vi "Run.vi"(8 "error in (no error)":errorcluster, 11 "RoomAlert in":refnum<class "RoomAlert.lvclass">) -> (0 "error out":errorcluster, 1 "DataValid":bool, 2 "clSensorData":T1, 3 "RoomAlert out":refnum<class "RoomAlert.lvclass">)   [LabVIEW 2018, in "SensorPlugins.lvlib" / "RoomAlert.lvclass"]
doc: "Retrieves measurements from the RoomAlert instrument."
uses:
  RoomAlert.lvclass
  SensorShared/clSensorData.ctl
  SensorShared/SensorVisulization.ctl
  <vilib>/Utility/error.llb/Error Cluster From Error Code.vi
  <vilib>/ErrorRing/Error Ring.xnode
  SensorShared/SensorShared.lvlib
panel:
  out "Execution Time (ms)":u32
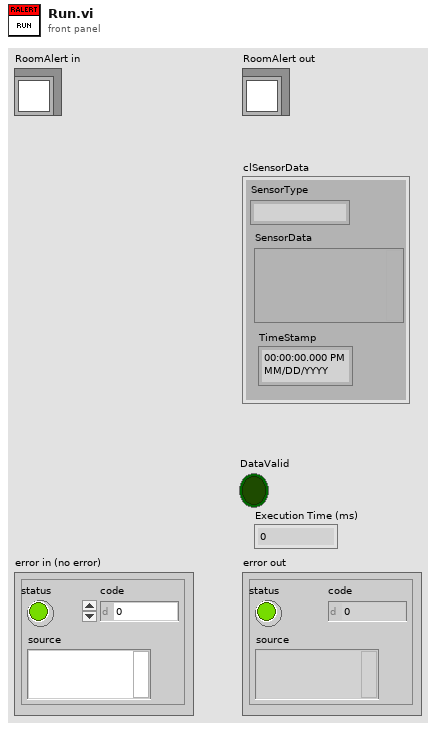
[diagram p1: front panel]
types:
  T1 = typedef "SensorShared.lvlib/clSensorData.ctl" = cluster{"SensorType":string, "SensorData":variant, "TimeStamp":timestamp}
  T2 = typedef "SensorShared.lvlib/SensorVisulization.ctl" = cluster{"Array of Waveforms":waveform(dbl)[], "Array of Strings ":string[], "LightTower":cluster{"Red":bool, "Amber":bool, "Green":bool, "Audio":bool}}
  T3 = typedef "SensorPlugins.lvlib/RoomAlert.lvclass/RoomAlertControls.ctl" = cluster{"Connected?":bool, "IP Address of SNMP Device":string, "Port (161)":u16, "Community Name":string, "Measurements To Read Array":u16[], "Update LightTower?":bool, "LightTower":cluster{"Red":bool, "Amber":bool, "Green":bool, "Audio":bool}, "RoomAlert Model ID":string, "Sensor OID Numbers":string[][], "Sensor Light Tower OID Numbers":string[][]}[]
  T4 = typedef "SensorPlugins.lvlib/RoomAlert.lvclass/CommunicationControls.ctl" = refnum<k16>[]
  T5 = typedef "SensorPlugins.lvlib/RoomAlert.lvclass/MeasurementControls.ctl" = cluster{"Measurement RefreshTime (ms)":u32, "Measurement Name":string, "Timeout(ms)":i32, "Amber Warning Light Configuration":cluster{"Warning Temperture (Degrees C)":dbl, "Temperature Delta (Degrees C/Minute)":dbl, "Time Window (Minutes)":dbl}}
  T6 = cluster{"Warning Temperture (Degrees C)":dbl, "Temperature Delta (Degrees C/Minute)":dbl, "Time Window (Minutes)":dbl}
  T7 = cluster{"[0]":bool, "[1]":bool, "[2]":bool, "[3]":bool}
  T8 = cluster{"Connected?":bool, "IP Address of SNMP Device":string, "Port (161)":u16, "Community Name":string, "Measurements To Read Array":u16[], "Update LightTower?":bool, "LightTower":cluster{"Red":bool, "Amber":bool, "Green":bool, "Audio":bool}, "RoomAlert Model ID":string, "Sensor OID Numbers":string[][], "Sensor Light Tower OID Numbers":string[][]}
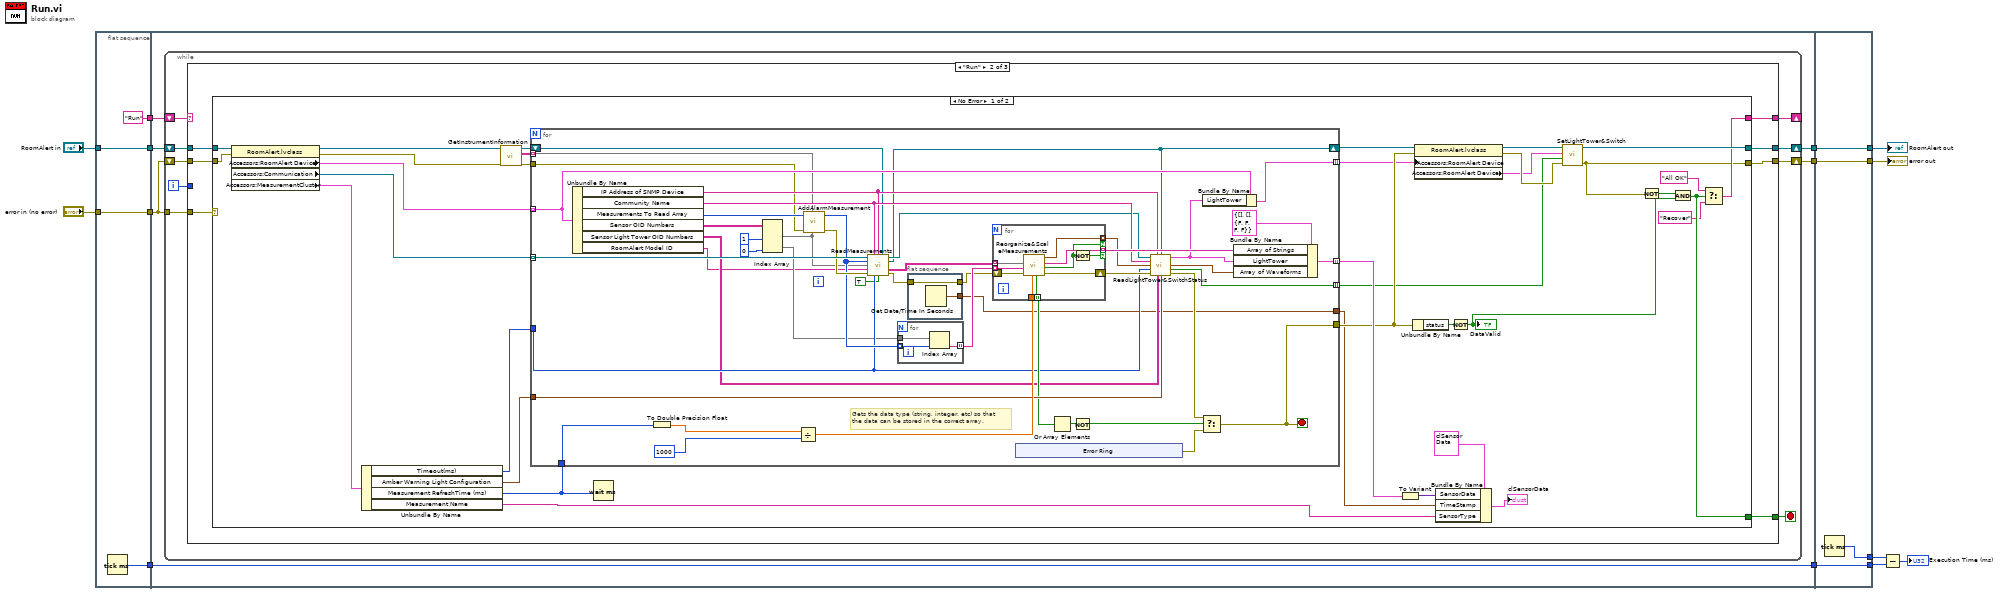
[diagram p0: block diagram]
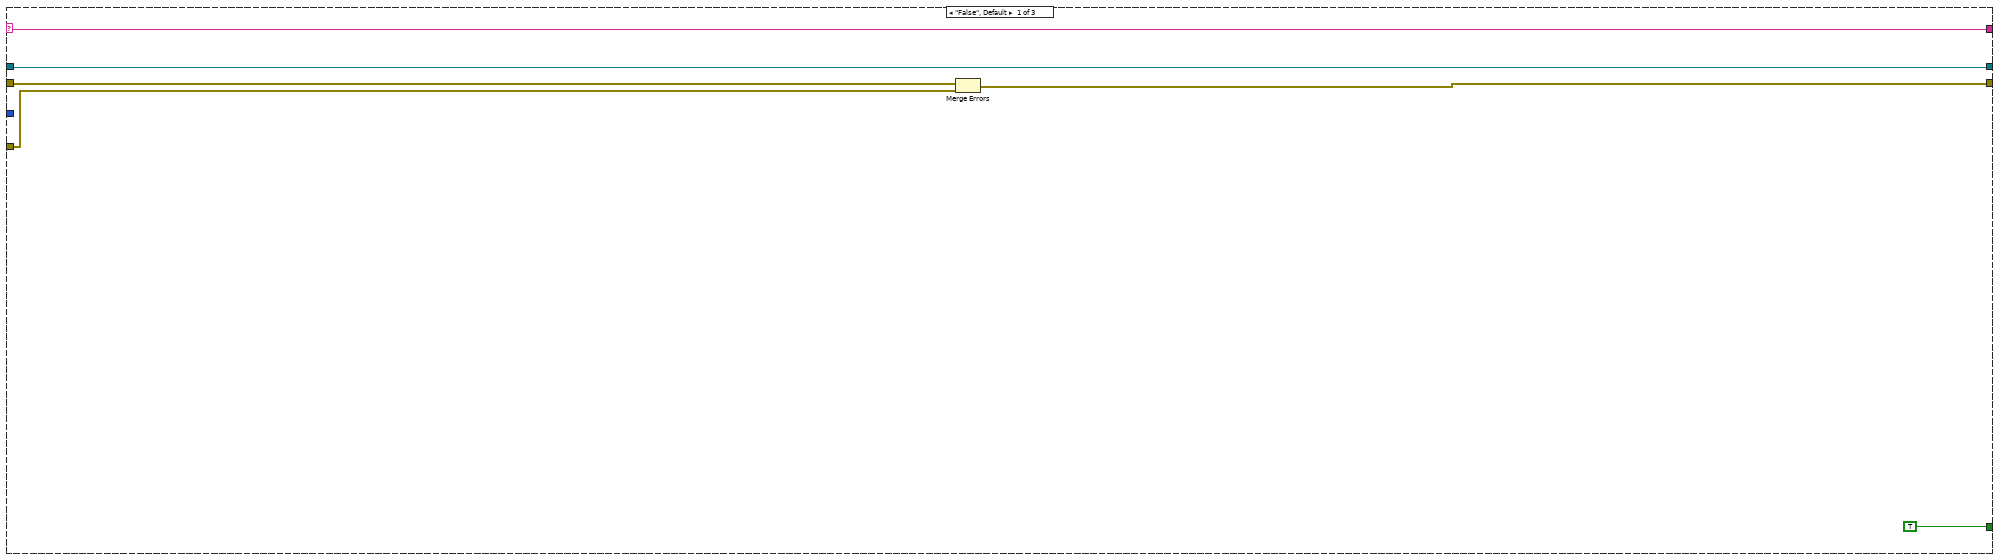
[diagram p2: hidden frame]
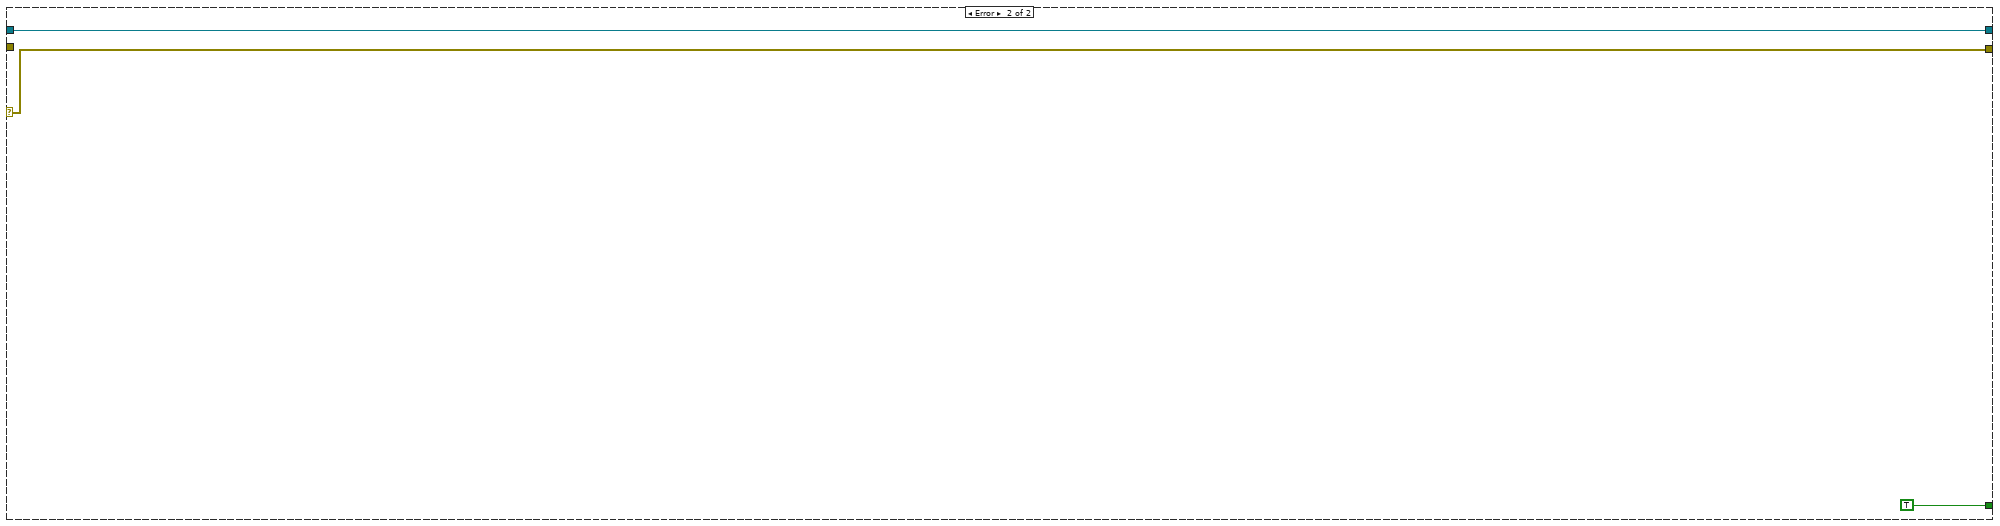
[diagram p3: hidden frame]
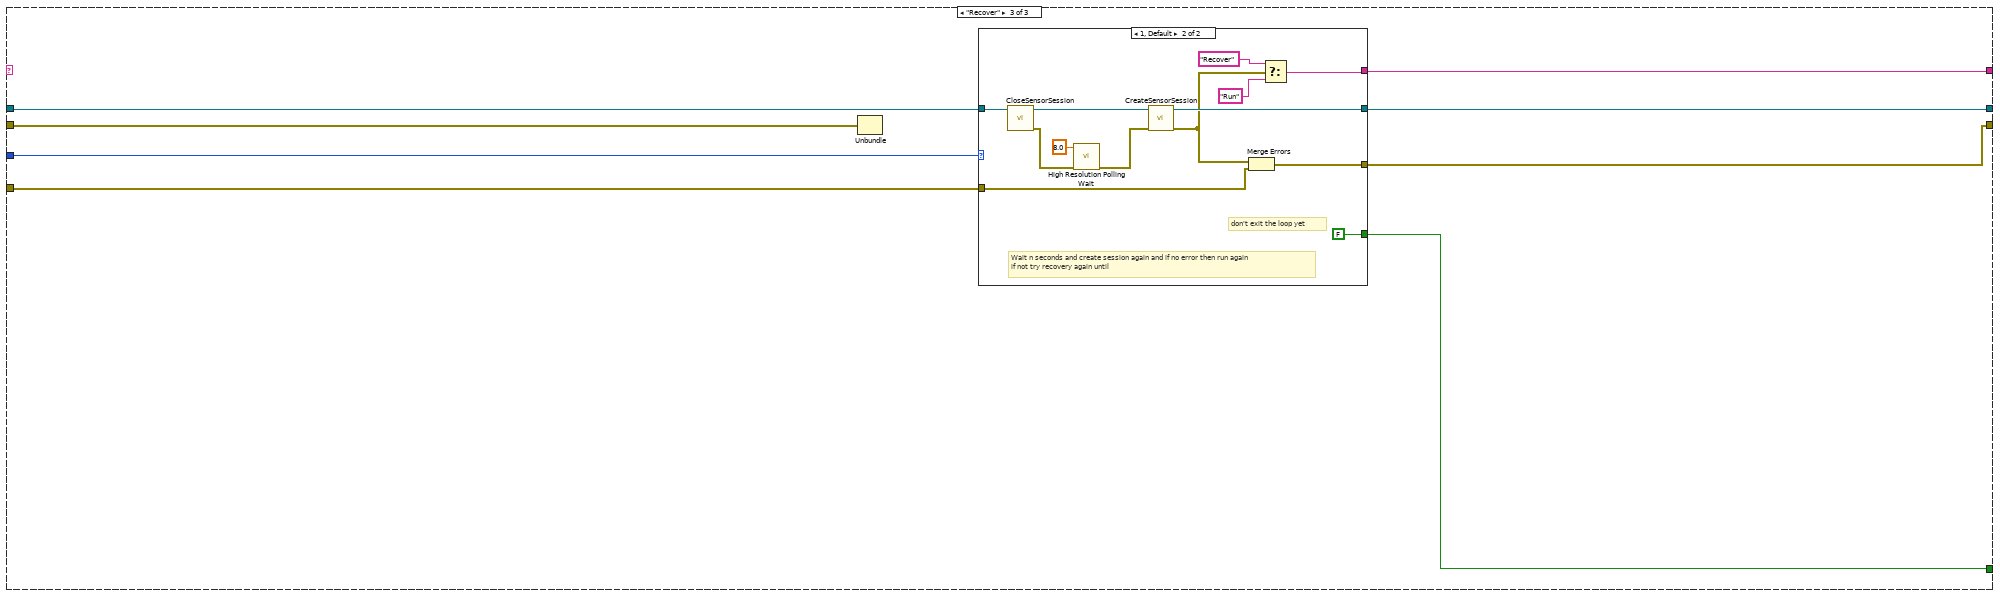
[diagram p4: hidden frame]
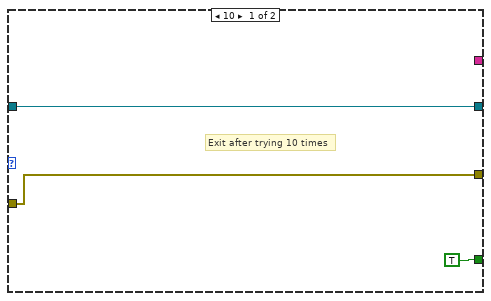
[diagram p5: hidden frame]
diagram:
  n1 = flat-sequence {
    tunnel: "RoomAlert in" -> [w17]
    tunnel: "error in (no error)" -> [w18]
    tunnel: [w18] -> w14
    tunnel: [w17] -> w13
    tunnel: [w16] -> w12
    tunnel: ["Run" ("Measurement Name")] -> w1
    tunnel: w14 -> [w19]
    tunnel: w13 -> [w24]
    tunnel: [w23] -> w9
    tunnel: [w22] -> w10
    tunnel: w12 -> [w21]
    tunnel: [w21] -> w11
    tunnel: w1 -> [w20]
    tunnel: [w177] -> w5
    tunnel: [w178] -> w6
    tunnel: w11 -> [w175]
    tunnel: w10 -> [w177]
    tunnel: w9 -> [w178]
    tunnel: [w176] -> w3
    tunnel: [w175] -> w2
    frame #0 {
      n2 = Tick Count (ms)() -> (millisecond timer value=w16:u32)
    }
    frame #1 {
      n3 = while {
        shift-right: [w30] -> w22
        shift-left: w19 -> [w33]
        shift-right: [w31] -> w23
        shift-left: w24 -> [w32]
        shift-right: [w28] -> _
        shift-left: w20 -> [w29]
        tunnel: w19 -> [w26]
        i -> [w25]
        stop <- w27 stop-if-true
        n4 = case shown="\"Run\"" w29 {
          selector: w29 -> [w39 _ _]
          tunnel: w33 -> [w37 w40 w151]
          tunnel: w32 -> [w38 w46 w158]
          tunnel: [w38 w45 w157] -> w31
          tunnel: [w36 w44 w153] -> w30
          tunnel: [w39 w43 w156] -> w28
          tunnel: [TRUE w42 w154] -> w27
          tunnel: w26 -> [w35 w41 w152]
          tunnel: w25 -> [_ _ w155]
          frame "False", Default {
            n5 = Merge Errors(w37, w35) -> (w36:errorcluster)
          }
          frame "Run" {
            n6 = case shown="No Error" w41 {
              selector: w41 -> [_ w150]
              tunnel: w46 -> [w81 w149]
              tunnel: [w52 w150] -> w44
              tunnel: [w69 w149] -> w45
              tunnel: [w55 _] -> w43
              tunnel: [w54 TRUE] -> w42
              tunnel: w40 -> [w53 _]
              frame No Error {
                n7 = property class="RoomAlert.lvclass"(reference=w81, error in=w53) -> (reference out=w65:refnum<class "RoomAlert.lvclass">, error out=w63:errorcluster, "Accessors:RoomAlert Device"=w57:T3, "Accessors:Communication "=w75:T4, "Accessors:MeasurementCluster"=w74:T5)
                n8 = Unbundle By Name(w74) -> ("Timeout(ms)"=w59:i32, "Amber Warning Light Configuration"=w58:T6, "Measurement RefreshTime (ms)"=w60:u32, "Measurement Name"=w48:string)
                n9 = call "GetInstrumentInformation.vi"("error in (no error)"=w63, "RoomAlert in"=w65) -> ("error out"=w62:errorcluster, "Model IDs"=w61:string[][][], "RoomAlert out"=w64:refnum<class "RoomAlert.lvclass">)  [unwired: 7 in]
                n10 = for {
                  tunnel: w57 -> [w101] mode=indexing
                  tunnel: [w111] -> w72
                  tunnel: [w127] -> w77 mode=indexing
                  tunnel: w75 -> [w126] mode=indexing
                  tunnel: w58 -> [w116]
                  tunnel: [w109] -> w68 mode=indexing
                  shift-right: [w85] -> w73
                  shift-left: w64 -> [w86]
                  tunnel: [w103] -> w66 mode=indexing
                  tunnel: w62 -> [w95]
                  tunnel: w61 -> [w98] mode=indexing
                  tunnel: w59 -> [w97]
                  tunnel: w60 -> [w96]
                  tunnel: [w82] -> w47
                  stop <- w111 stop-if-true
                  # "Gets the data type (string, integer, etc) so that\nthe data can be stored in the correct array."
                  n11 = Unbundle By Name(w101) -> ("IP Address of SNMP Device"=w118:string, "Community Name"=w119:string, "Measurements To Read Array"=w102:u16[], "Sensor OID Numbers"=w94:string[][], "Sensor Light Tower OID Numbers"=w89:string[][], "RoomAlert Model ID"=w87:string)
                  n12 = To Double Precision Float(number=w96) -> (double precision float=w124:dbl)
                  n13 = Index Array(array=w94, index (col) #1=1 ("disabled index (col)"), index (col) #2=0 ("index (col)")) -> (element #1=w92:string[], element #2=w90:string[])  [unwired: 2 in]
                  n14 = Divide(x=w124, y=u32 1000) -> (x/y=w122:dbl)
                  n15 = call "AddAlarmMeasurement.vi"("OID Numbers"=w92, "Model Information"=w98, "Error In"=w95, "Measurements To Read Array In"=w102) -> ("Error Out"=w100:errorcluster, "Measurements To Read Array Out"=w99:u16[])  [unwired: 6 in]
                  n16 = call "ReadMeasurements.vi"("UDP Network Connection in"=w126, "Community Name"=w119, "IP Address of SNMP Device"=w118, "RoomAlert in"=w86, "Measurements To Read Array"=w99, "OID Numbers"=w92, "Instrument Model ID"=w87, "error in (no error)"=w100, "Timeout(ms)"=w97, "Filter OID Numbers? (T)"=TRUE) -> ("UDP Network Connection out"=w106:refnum<k16>, "RoomAlert Out"=w85:refnum<class "RoomAlert.lvclass">, "SNMPDataAsStrings"=w117:string[][], "error out"=w84:errorcluster)  [unwired: 2 in]
                  n17 = for {
                    tunnel: w99 -> [w136] mode=indexing
                    tunnel: w90 -> [w137]
                    tunnel: [w135] -> w120 mode=indexing
                    n18 = Index Array(array=w137, index=w136) -> (element=w135:string)
                  }
                  n19 = flat-sequence {
                    tunnel: w84 -> [w129]
                    tunnel: [w129] -> w83
                    tunnel: [w128] -> w82
                    frame #0 {
                      n20 = Get Date/Time In Seconds() -> (seconds since 1Jan1904=w128:timestamp)
                    }
                  }
                  n21 = for {
                    tunnel: w117 -> [w138] mode=indexing
                    shift-right: [w146] -> w108
                    shift-left: w83 -> [w147]
                    tunnel: [w145] -> w105 mode=indexing if=w142
                    tunnel: w122 -> [w141]
                    tunnel: [w144] -> w123 mode=indexing if=w143
                    tunnel: w120 -> [w139] mode=indexing
                    tunnel: [w140] -> w115 mode=indexing
                    n22 = call "Reorganize&ScaleMeasurements.vi"("Meas Aperature"=w141, "Error In"=w147, "MeasurementType"=w139, "SNMPDataAsStrings"=w138) -> ("Error Out"=w146:errorcluster, "Numerical Information"=w142:bool, "String Data"=w144:string, "output waveform"=w145:waveform(dbl), "Alarmed"=w140:bool)  [unwired: 3 in]
                    n23 = Not(x=w142) -> (.not. x?=w143:bool)
                  }
                  n24 = xnode "Error Ring"() -> ("error out"=w114:errorcluster)
                  n25 = Or Array Elements(Boolean array=w115) -> (logical OR=w113:bool)
                  n26 = Not(x=w113) -> (.not. x?=w112:bool)
                  n27 = call "ReadLightTower&SwitchStatus.vi"("UDP Network Connection in"=w106, "IP Address of SNMP Device"=w118, "RoomAlert in"=w85, "Community Name"=w119, "Array In"=w105, "Timeout(ms)"=w97, "error in (no error)"=w108, "LightTower OID"=w89, "Amber Warning Light Limits"=w116) -> ("Light Tower"=w110:T7, "Array Out"=w104:waveform(dbl)[], "Yellow Limit Exceeded?"=w103:bool, "error out"=w107:errorcluster)  [unwired: 3 in]
                  n28 = Select(t=w107, s=w112, f=w114) -> (s? t:f=w111:errorcluster)
                  n29 = Bundle By Name(cluster=w101, "LightTower"=w110) -> (w109:T8)
                  n30 = Bundle By Name(cluster=T2 {"Array of Waveforms"=[], "Array of Strings "=[], "LightTower"={"Red"=FALSE, "Amber"=FALSE, "Green"=FALSE, "Audio"=FALSE}} ("SiemensDEMMeasurements 2"), "Array of Strings"=w123, "LightTower"=w110, "Array of Waveforms"=w104) -> (w127:T2)
                }
                n31 = Wait (ms)(milliseconds to wait=w60) -> ()  [unwired: 1 out]
                n32 = To Variant(anything=w77) -> (Variant=w79:variant)
                n33 = Unbundle By Name(w72) -> ("status"=w78:bool)
                n34 = property class="RoomAlert.lvclass"(reference=w73, error in=w72, "Accessors:RoomAlert Device"=w68) -> (reference out=w70:refnum<class "RoomAlert.lvclass">, error out=w71:errorcluster, "Accessors:RoomAlert Device"=w67:T3)
                n35 = Bundle By Name(cluster=T1 {"SensorType"="", "SensorData"=variant, "TimeStamp"=timestamp(0 s since 1904-01-01)} ("clSensorData"), "SensorData"=w79, "TimeStamp"=w47, "SensorType"=w48) -> (→"clSensorData":T1)
                n36 = Not(x=w78) -> (.not. x?=w56:bool)
                "DataValid" <- w56
                n37 = call-dynamic "SetLightTower&Switch.vi"("error in (no error)"=w71, "UpdateValue? (F)"=w66, "RoomAlert Device"=w67, "RoomAlert in"=w70) -> ("error out"=w52:errorcluster, "RoomAlert out"=w69:refnum<class "RoomAlert.lvclass">)  [unwired: 6 in]
                n38 = Not(x=w52) -> (.not. x?=w49:bool)
                n39 = And(x=w49, y=w56) -> (x .and. y?=w54:bool)
                n40 = Select(t="All OK", s=w54, f="Recover" ("Measurement Name")) -> (s? t:f=w55:string)
              }
              frame Error {
              }
            }
          }
          frame "Recover" {
            n41 = Unbundle(w151) -> ()  [unwired: 3 out]
            n42 = case shown="1, Default" w155 {
              tunnel: w158 -> [w161 w174]
              tunnel: [w161 w169] -> w157
              tunnel: [_ w166] -> w156
              tunnel: [TRUE FALSE] -> w154
              tunnel: w152 -> [w159 w163]
              tunnel: [w159 w162] -> w153
              frame 10 {
                # "Exit after trying 10 times"
              }
              frame 1, Default {
                # "don't exit the loop yet"
                # "Wait n seconds and create session again and if no error then run again\nif not try recovery again until"
                n43 = call-dynamic "CloseSensorSession.vi"("RoomAlert in"=w174) -> ("error out"=w173:errorcluster, "RoomAlert out"=w171:refnum<class "RoomAlert.lvclass">)  [unwired: 9 in]
                n44 = call <vilib>:"High Resolution Polling Wait.vi"("error in (no error)"=w173, "seconds to wait"=8.0) -> ("error out"=w170:errorcluster)  [unwired: 9 in]
                n45 = call-dynamic "CreateSensorSession.vi"("error in (no error)"=w170, "RoomAlert in"=w171) -> ("error out"=w164:errorcluster, "RoomAlert out"=w169:refnum<class "RoomAlert.lvclass">)  [unwired: 8 in]
                n46 = Merge Errors(w164, w163) -> (w162:errorcluster)
                n47 = Select(t="Recover" ("Measurement Name"), s=w164, f="Run" ("Measurement Name")) -> (s? t:f=w166:string)
              }
            }
          }
        }
      }
    }
    frame #2 {
      n48 = Tick Count (ms)() -> (millisecond timer value=w176:u32)
    }
  }
  n49 = Subtract(x=w3, y=w2) -> (x-y=→"Execution Time (ms)":u32)
  "error out" <- w5
  "RoomAlert out" <- w6
